vi "Day 4 main.vi"() -> ()   [LabVIEW 2020]
uses:
  bf0b99a3-431b-4a45-be7d-e08dca16cb5f.vi
panel:
  out "Any overlap":i32
  out "Completely overlap":i32
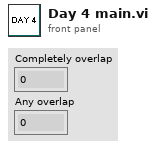
[diagram p1: front panel]
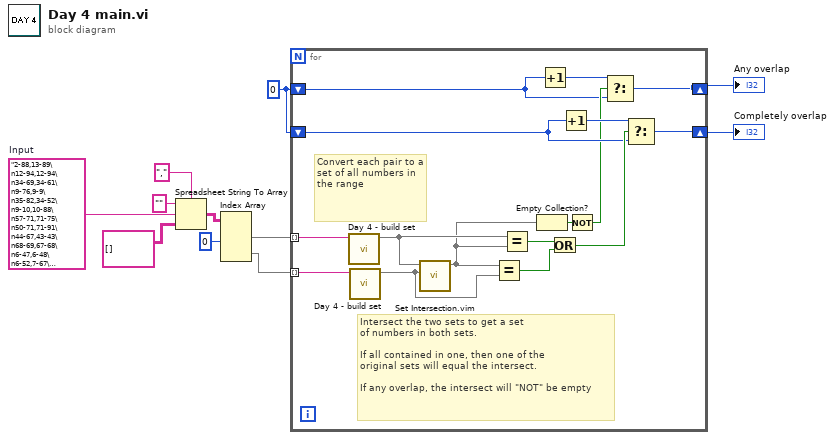
[diagram p0: block diagram]
diagram:
  w2 = 0
  w11 = "2-88,13-89\n12-94,12-94\n34-69,34-61\n9-76,9-9\n35-82,34-52\n9-10,10-88\n57-71,71-75\n50-71,71-91\n44-67,43-43\n68-69,67-68\n6-47,6-48\n6-52,7-67\n43-51,40-44\n56-67,57-69\n94-94,68-94\n10-97,9-9\n40-95,40-98\n22-81,22-22\n7-58,7-59\n8-82,82-82\n22-27,23-44\n5-27,7-28\n11-75,11-75\n7-90,99-99\n65-89,65-66\n24-52,29-53\n41-57,27-58\n14-95,13-26\n27-34,26-75\n18-33,33-56\n21-95,21-95\n20-29,69-71\n81-81,23-90\n47-83,47-82\n28-50,86-98\n50-76,21-50\n3-69,64-79\n17-97,10-16\n54-92,10-93\n7-75,45-77\n72-72,42-73\n13-80,81-87\n25-26,25-64\n38-48,38-38\n2-99,2-99\n48-93,67-92\n12-85,2-94\n14-75,7-82\n29-46,23-29\n50-94,4-51\n3-37,37-91\n24-91,91-91\n25-48,44-47\n2-77,1-26\n1-58,1-21\n16-93,16-93\n3-99,8-98\n23-23,6-23\n17-67,68-68\n4-15,1-4\n35-41,35-40\n6-88,52-89\n11-48,11-61\n4-64,12-65\n7-90,7-8\n1-89,6-73\n64-69,38-70\n26-67,59-66\n41-54,16-42\n2-99,9-96\n2-8,7-88\n12-95,97-97\n17-92,12-93\n27-56,27-28\n19-66,65-77\n1-95,94-94\n24-48,23-95\n40-74,74-74\n20-99,20-97\n60-73,61-74\n23-85,23-86\n37-69,69-69\n37-64,27-37\n7-53,7-27\n84-97,93-94\n26-51,50-52\n12-93,13-93\n28-86,29-29\n11-25,18-46\n97-99,91-98\n27-73,53-58\n25-77,6-26\n26-29,29-68\n11-17,11-28\n99-99,13-99\n70-92,48-92\n50-61,50-62\n2-95,77-94\n17-17,17-90\n95-95,16-95\n12-96,13-97\n28-98,28-28\n18-91,3-80\n1-95,1-19\n86-89,22-89\n37-96,3-96\n2-18,18-56\n8-72,71-73\n46-48,32-47\n57-69,57-78\n10-22,9-9\n6-96,6-6\n44-58,5-59\n6-8,7-93\n76-95,77-99\n97-99,3-98\n69-69,64-69\n38-68,67-96\n68-74,67-95\n20-68,69-69\n6-88,9-85\n47-66,47-55\n9-94,93-95\n19-29,28-89\n4-83,90-90\n2-95,1-95\n36-37,36-36\n12-90,45-68\n1-80,89-94\n95-99,6-96\n1-1,2-95\n47-81,46-80\n1-57,38-47\n5-7,7-98\n18-75,18-94\n39-70,39-70\n62-93,62-62\n30-32,31-54\n22-82,82-84\n83-92,84-98\n54-93,6-94\n74-91,73-90\n11-90,11-90\n92-98,96-97\n13-73,55-69\n47-95,46-95\n11-97,11-99\n53-68,53-53\n45-89,45-46\n99-99,38-89\n14-88,96-96\n6-78,6-7\n31-67,67-67\n96-96,48-96\n40-69,25-39\n10-60,9-61\n38-97,78-93\n52-69,51-60\n21-72,21-33\n24-90,89-90\n36-83,84-84\n44-58,44-68\n95-95,82-94\n13-91,91-95\n27-95,94-96\n60-82,61-83\n11-77,12-12\n7-91,6-90\n15-94,14-48\n5-73,5-74\n10-40,10-40\n59-94,59-93\n84-84,84-84\n8-8,7-75\n20-81,20-81\n5-96,96-99\n5-63,5-6\n2-93,2-93\n72-74,31-73\n6-54,5-47\n8-36,9-86\n1-95,94-94\n11-66,10-73\n45-52,52-99\n1-92,1-95\n76-90,76-77\n6-53,54-55\n44-52,45-95\n5-70,27-70\n3-56,6-55\n28-37,36-37\n54-97,54-98\n4-63,1-4\n5-64,65-65\n19-74,17-18\n12-26,12-12\n34-78,35-99\n42-42,3-42\n69-70,69-77\n49-75,50-95\n30-52,1-28\n25-80,25-25\n97-99,10-98\n36-55,36-54\n6-55,8-55\n60-80,61-81\n76-81,37-77\n19-20,20-20\n11-33,33-85\n31-60,7-32\n3-9,1-2\n40-87,22-40\n9-35,8-35\n9-75,35-75\n19-86,18-85\n33-52,45-53\n15-49,49-66\n40-83,1-41\n10-54,23-88\n83-94,43-83\n7-74,3-75\n18-79,17-18\n6-63,1-6\n19-39,39-77\n69-78,69-79\n14-26,1-23\n3-49,1-58\n39-40,38-39\n16-58,54-57\n34-83,17-34\n79-88,10-80\n73-86,73-86\n4-15,13-14\n6-94,6-6\n84-93,35-84\n56-81,55-81\n3-30,3-4\n5-94,4-96\n5-87,42-87\n98-99,63-79\n20-95,10-21\n40-87,39-41\n39-90,40-97\n20-54,24-88\n1-40,2-65\n57-97,63-96\n1-42,1-1\n5-11,11-66\n39-96,38-95\n5-72,6-73\n7-7,10-96\n97-97,13-97\n71-97,2-4\n79-79,76-79\n20-56,56-74\n57-76,62-68\n20-63,20-57\n19-68,69-69\n41-70,41-70\n37-42,27-44\n77-98,57-99\n18-92,91-96\n10-85,10-96\n43-61,6-44\n25-65,66-95\n12-29,12-80\n22-70,69-71\n77-78,6-77\n20-89,22-88\n79-88,20-88\n98-98,3-99\n58-80,58-66\n27-32,25-47\n80-91,80-95\n24-70,24-86\n52-60,52-62\n80-80,16-80\n3-43,10-88\n2-80,1-99\n34-87,34-88\n28-30,28-32\n13-55,7-55\n16-38,7-16\n25-33,32-77\n58-90,57-57\n7-94,6-7\n5-97,32-96\n71-71,51-71\n10-21,10-11\n3-9,8-98\n26-34,1-81\n35-49,35-50\n11-70,10-71\n25-72,24-99\n27-84,71-72\n50-72,50-71\n11-62,11-34\n93-97,92-96\n71-71,28-71\n72-80,65-81\n27-32,23-28\n31-79,32-79\n12-80,12-81\n38-63,6-39\n27-98,60-97\n45-83,35-45\n52-52,30-52\n11-97,12-14\n3-94,1-99\n4-23,16-22\n1-12,13-91\n14-80,14-78\n3-89,1-3\n28-99,27-87\n14-50,11-66\n40-88,39-39\n38-98,98-99\n5-91,4-91\n4-22,23-23\n20-90,24-91\n2-63,1-62\n14-81,13-80\n52-52,1-51\n8-11,11-93\n9-66,1-9\n44-86,43-68\n13-13,13-94\n40-67,40-68\n70-73,34-68\n5-83,2-11\n37-49,36-49\n11-97,99-99\n44-99,43-98\n50-98,50-97\n38-39,38-80\n83-83,2-84\n14-40,3-23\n41-94,41-96\n61-83,59-62\n22-95,22-96\n32-77,32-77\n22-97,23-96\n39-85,70-84\n4-95,3-95\n14-39,14-38\n9-68,68-96\n62-63,3-48\n21-25,22-90\n4-4,3-98\n85-89,85-99\n7-42,7-43\n31-82,82-84\n45-53,41-54\n38-66,37-66\n5-80,4-72\n1-1,2-97\n3-3,2-3\n47-61,42-61\n70-94,94-98\n1-51,1-51\n53-70,93-99\n43-72,72-82\n3-7,6-77\n71-95,82-92\n82-89,6-82\n3-43,4-76\n45-91,46-91\n12-87,13-87\n11-92,11-46\n3-73,3-72\n91-91,47-92\n12-93,14-94\n43-45,9-44\n10-87,11-87\n20-34,33-88\n48-71,15-97\n20-64,19-64\n3-57,57-57\n6-7,7-99\n4-19,19-96\n68-72,69-72\n14-45,14-14\n22-93,22-23\n8-34,8-15\n83-93,92-96\n11-94,12-94\n54-84,38-85\n93-98,3-55\n32-77,39-40\n3-15,15-93\n16-28,11-29\n1-95,94-96\n6-25,25-26\n32-96,99-99\n1-35,2-5\n73-91,65-74\n62-77,41-63\n72-72,72-93\n5-81,5-81\n81-83,32-81\n68-89,68-89\n30-35,30-61\n48-97,8-49\n85-94,12-94\n15-95,15-96\n4-98,3-4\n33-84,33-92\n28-58,29-59\n44-80,44-80\n11-84,83-83\n95-98,1-96\n3-44,21-43\n91-91,46-69\n91-98,1-90\n3-20,19-72\n3-92,4-55\n23-68,98-98\n26-97,80-83\n98-98,2-97\n30-92,74-92\n6-44,7-60\n18-23,36-47\n9-94,98-99\n11-20,11-75\n50-95,5-51\n13-83,20-84\n27-27,27-47\n95-96,56-95\n27-28,27-29\n31-95,31-31\n19-50,21-23\n19-48,30-55\n7-36,22-80\n3-5,6-99\n21-22,23-52\n3-70,3-70\n4-8,7-90\n28-60,60-98\n81-93,58-82\n2-6,3-16\n15-75,16-76\n8-86,6-6\n1-78,78-95\n37-91,37-99\n94-94,17-94\n53-80,80-81\n1-90,89-89\n21-32,21-73\n65-74,65-74\n24-54,89-92\n8-47,9-47\n8-36,12-41\n6-79,1-23\n79-83,24-84\n91-91,16-92\n14-84,14-15\n51-67,50-50\n6-93,96-96\n29-55,29-43\n36-37,36-77\n36-36,19-35\n84-84,60-89\n66-88,14-89\n14-69,28-93\n79-94,39-62\n85-89,89-89\n1-78,2-78\n44-52,42-53\n55-97,55-97\n32-81,74-80\n90-90,16-89\n3-96,2-37\n15-58,16-71\n5-93,6-93\n1-4,4-13\n61-96,61-99\n17-87,17-86\n34-48,35-49\n17-58,10-17\n1-11,12-68\n56-86,27-64\n73-80,73-77\n96-96,76-97\n23-32,23-31\n3-94,5-95\n67-98,66-72\n87-93,56-92\n4-15,5-15\n24-76,25-75\n43-59,33-60\n66-74,66-68\n18-90,17-57\n68-72,72-93\n6-19,19-29\n94-99,6-95\n20-85,10-21\n45-66,45-67\n73-74,12-73\n35-75,34-59\n67-88,80-88\n99-99,2-97\n15-90,14-14\n9-59,9-86\n18-52,52-79\n65-73,27-74\n89-96,88-96\n97-97,5-78\n92-94,48-93\n27-40,27-57\n7-95,1-8\n7-17,7-49\n66-66,65-89\n7-46,12-78\n15-29,15-38\n7-7,8-64\n13-22,13-21\n11-11,10-45\n84-84,30-84\n42-91,91-91\n65-87,29-87\n87-87,18-86\n17-66,17-65\n87-88,78-86\n57-57,58-87\n22-53,22-54\n8-62,7-62\n37-90,37-91\n50-86,49-86\n6-58,6-67\n32-60,32-63\n91-96,91-91\n13-94,13-14\n4-95,4-95\n1-86,4-87\n30-96,59-95\n10-28,8-59\n2-49,66-71\n96-99,4-97\n3-74,2-2\n29-76,75-75\n4-92,4-91\n16-94,14-16\n35-35,36-96\n39-67,66-66\n17-97,16-67\n1-99,46-98\n41-74,40-74\n45-68,45-69\n68-95,94-99\n14-51,13-31\n91-91,4-91\n46-66,2-67\n61-66,6-71\n66-69,55-89\n11-11,6-10\n72-91,73-94\n1-92,1-16\n25-98,35-74\n56-87,73-87\n57-59,1-58\n4-5,4-91\n27-31,30-68\n98-98,22-98\n28-95,84-94\n9-24,8-24\n21-30,22-38\n79-81,6-83\n34-96,34-83\n31-33,26-32\n36-59,50-52\n25-95,19-25\n97-97,75-90\n97-99,27-98\n7-48,32-52\n12-72,11-33\n3-41,3-41\n2-95,3-95\n71-71,52-72\n92-98,20-92\n14-90,15-99\n86-97,85-87\n44-71,44-71\n10-68,1-10\n47-77,11-46\n8-25,25-47\n22-34,25-34\n17-90,18-48\n31-94,30-94\n10-97,10-96\n21-44,22-97\n42-97,2-98\n84-91,50-85\n60-96,78-82\n81-85,73-80\n41-73,40-73\n48-65,47-56\n5-42,6-79\n33-33,33-83\n46-79,47-79\n61-91,23-92\n93-95,3-94\n32-43,31-51\n83-97,70-83\n24-93,94-94\n2-94,8-91\n45-61,46-65\n46-50,48-75\n23-95,57-84\n3-99,92-95\n85-85,2-61\n42-87,87-93\n95-99,2-96\n3-4,3-98\n1-87,7-87\n34-72,72-73\n11-84,8-12\n80-99,63-98\n96-99,7-97\n73-75,30-73\n60-87,7-61\n21-41,19-40\n14-77,76-86\n53-97,36-98\n34-54,33-54\n4-36,11-66\n6-10,10-94\n1-57,3-87\n15-39,16-39\n34-72,14-33\n1-3,3-93\n23-53,22-53\n24-44,23-34\n9-28,3-9\n12-99,99-99\n87-98,87-98\n11-11,11-73\n96-96,4-91\n91-91,8-92\n18-47,18-94\n57-59,27-59\n12-96,13-75\n1-27,26-61\n21-60,60-61\n30-67,31-67\n22-78,22-78\n6-77,7-52\n28-45,44-78\n34-87,90-94\n65-76,77-77\n11-76,57-58\n83-84,14-83\n70-97,11-70\n97-98,11-97\n29-29,16-29\n87-94,18-87\n53-71,70-70\n3-96,2-90\n11-80,13-99\n68-68,69-83\n64-97,1-98\n39-42,40-58\n35-49,35-49\n58-88,58-87\n67-67,13-66\n20-20,6-19\n16-67,16-17\n3-46,2-4\n41-96,41-88\n20-89,18-21\n4-84,4-84\n81-82,20-81\n94-94,28-93\n64-74,8-65\n3-73,5-36\n15-67,6-86\n33-33,32-91\n23-97,57-97\n8-58,8-46\n9-10,9-99\n67-93,69-92\n93-99,5-93\n95-96,95-98\n15-22,35-53\n55-97,38-98\n95-99,3-96\n12-12,12-62\n89-89,41-88\n9-10,9-92\n41-85,67-84\n10-97,2-11\n19-73,61-72\n38-79,78-80\n49-61,50-72\n70-71,71-72\n25-32,26-31\n2-5,3-62\n12-94,11-93\n26-95,27-98\n40-81,40-80\n34-71,34-95\n99-99,16-89\n14-93,93-96\n19-70,4-20\n7-28,1-29\n13-59,12-59\n44-97,11-45\n8-36,36-37\n94-95,7-94\n43-43,9-42\n16-98,3-13\n89-96,59-82\n9-50,9-51\n70-98,69-97\n84-87,84-87\n25-83,13-70\n63-71,62-71\n3-31,3-96\n53-67,13-76\n98-98,59-99\n4-39,5-40\n19-91,17-90\n28-50,36-45\n34-86,33-38\n58-80,57-80\n90-90,9-90\n98-98,37-72\n2-39,3-53\n85-97,28-84\n96-97,86-98\n38-78,30-39\n1-42,2-41\n7-28,8-27\n6-74,7-75\n85-87,49-86\n98-98,16-46\n42-90,41-70\n5-70,6-70\n13-75,75-75\n25-69,5-51\n13-43,2-14\n77-91,78-78\n17-97,16-18\n3-94,1-3\n33-86,32-92\n13-57,57-68\n18-88,19-95\n11-97,11-96\n17-67,17-67\n44-95,44-94\n21-85,20-85\n30-64,41-64\n34-68,35-68\n37-77,77-79\n96-97,9-96\n78-85,9-79\n80-80,35-79\n16-50,16-36\n65-85,7-85\n52-92,2-52\n77-77,30-78\n4-61,2-5\n41-91,30-90\n93-96,20-90\n9-11,10-73\n39-42,38-42\n46-72,45-76\n57-63,56-66\n9-68,5-46\n5-92,98-98\n39-46,39-46\n10-48,10-65\n3-22,7-91\n43-82,2-94\n21-69,20-69\n70-70,2-71\n9-94,8-91\n23-99,23-80\n6-98,6-97\n45-45,22-44\n31-79,32-32\n47-67,47-48\n5-80,80-81\n34-54,29-55\n16-97,16-96\n6-71,71-74\n17-47,17-46\n74-85,85-86\n7-10,9-82\n30-30,30-90\n51-54,55-55\n20-28,21-98\n67-67,64-66\n50-51,35-50\n4-68,5-5\n1-4,4-40\n20-20,20-84\n29-31,26-73\n12-12,11-12\n45-94,44-93\n36-45,18-37\n14-41,13-98\n38-42,42-84\n32-63,31-62\n32-79,1-79\n32-32,32-88\n83-95,83-96\n50-84,49-83\n30-56,30-74\n7-67,67-82\n5-39,40-94\n3-7,7-82\n42-45,42-67\n1-97,96-99\n30-87,30-64\n3-97,3-98\n52-81,52-81\n65-80,65-80\n46-55,54-91\n17-88,87-92\n7-97,97-97\n57-81,57-81\n54-97,54-54\n13-13,13-86\n30-35,36-36\n77-77,68-76\n11-82,12-91\n7-72,2-48\n85-94,28-86\n17-88,88-99\n9-56,7-9\n56-96,33-96\n85-89,85-89\n13-13,13-99\n76-93,62-76\n86-86,31-86\n31-95,31-96\n68-70,44-69\n9-54,9-10\n66-97,25-98\n44-93,93-93\n63-63,17-62\n3-98,2-10\n18-96,19-97\n19-80,2-81\n44-45,4-44\n1-37,7-36\n59-61,39-62\n33-98,33-57\n38-77,37-76\n13-96,11-14\n28-98,29-99\n4-44,2-45\n37-95,37-95\n53-68,54-68\n3-72,4-88\n14-21,21-82\n43-65,42-47\n21-52,51-93\n65-79,56-65\n22-65,36-77\n42-54,53-99\n10-95,9-95\n1-78,2-76\n81-81,16-81\n26-49,29-70\n45-87,44-87\n14-15,14-67\n14-15,14-84\n2-42,41-79\n1-93,93-94\n61-98,60-97\n3-9,12-99\n48-62,49-56\n64-65,41-64\n27-52,27-51\n88-91,30-89\n17-46,46-46\n10-80,11-81\n3-7,1-6\n80-81,80-96\n67-96,67-96\n96-98,2-96\n89-90,60-89\n16-83,16-82\n67-77,68-70\n33-68,33-37\n8-29,1-7\n28-71,28-70\n64-89,79-89\n18-35,18-36\n20-86,20-88\n68-69,40-68\n24-74,23-82\n79-88,79-88\n5-56,4-55\n1-98,2-2\n10-99,4-24\n12-15,13-15\n30-93,99-99\n6-14,6-97\n3-86,4-52\n15-52,13-52\n28-78,78-79\n27-28,27-95\n40-88,29-96\n1-3,2-52\n27-43,27-33\n23-65,54-99\n4-49,48-50\n46-67,47-68\n94-94,2-94\n24-31,30-66\n14-87,6-58\n2-5,4-98\n40-92,39-91\n2-87,87-88\n7-74,19-73\n58-91,58-92\n11-82,5-97\n62-65,4-62\n95-96,8-95\n6-68,6-68\n5-98,4-10\n46-72,89-96\n24-58,58-92\n33-36,37-94\n47-48,48-76\n18-20,3-32\n11-65,10-58\n32-97,32-95\n27-53,19-75\n10-60,45-59\n32-62,63-65\n1-88,2-88\n48-93,63-92\n46-79,78-96\n18-47,4-17\n6-63,6-7\n39-80,36-69\n20-78,20-78\n26-81,26-27\n23-96,20-79\n45-59,45-60\n37-47,36-64\n33-45,5-42\n3-98,4-98\n18-75,4-19\n10-93,10-10\n24-70,7-24\n20-53,40-49\n56-81,72-80\n1-70,4-71\n15-18,19-92\n84-98,83-95\n35-48,47-49\n27-63,62-78\n9-79,14-95\n5-77,4-77\n20-39,20-40\n26-67,72-92\n69-80,55-80\n68-83,68-92\n87-87,6-86\n1-92,1-94\n14-81,14-99\n49-51,49-52\n71-71,49-70\n69-70,69-72\n18-54,3-50\n97-99,1-97\n4-34,33-33\n67-84,11-84\n31-52,47-51\n81-97,97-98\n27-62,54-61\n1-83,1-99\n30-78,30-78\n12-38,12-37\n37-76,24-74\n1-96,1-95\n96-96,12-96\n41-61,40-60\n81-87,81-99\n1-19,9-19\n2-8,7-42\n35-36,36-71\n67-79,67-78\n69-69,65-68\n8-8,9-64\n4-12,6-78\n14-47,47-64\n9-93,9-93\n95-98,15-29\n30-87,88-88\n12-77,78-78\n8-15,18-50\n10-98,11-97\n1-2,1-97\n2-92,2-86\n50-50,50-87"  # Input
  n1 = Spreadsheet String To Array(delimiter (Tab)=",", format string="", spreadsheet string=w11, array type (2D Dbl)=string[][] []) -> (array=w7:string[][])
  n2 = Index Array(array=w7, index (col) #1=0 ("disabled index (col)")) -> (element #1=w5:string[], element #2=w4:string[])  [unwired: 3 in]
  n3 = for {
    tunnel: w5 -> [w13] mode=indexing
    tunnel: w4 -> [w12] mode=indexing
    shift-right: [w23] -> w3
    shift-left: w2 -> [w20]
    shift-right: [w15] -> w1
    shift-left: w2 -> [w14]
    # "Intersect the two sets to get a set\nof numbers in both sets.\n\nIf all contained in one, then one of the \noriginal sets will equal the intersect.\n\nIf any overlap, the intersect will \"NOT\" be empty"
    # "Convert each pair to a set of all numbers in the range"
    n4 = call "Day 4 - build set.vi"("String (a-b)"=w13) -> ("Set (a..b inclusive)"=w27:set{i32})  [unwired: 10 in]
    n5 = call "Day 4 - build set.vi"("String (a-b)"=w12) -> ("Set (a..b inclusive)"=w26:set{i32})  [unwired: 10 in]
    n6 = call "Set Intersection.vim"("set 2"=w26, "set 1"=w27) -> ("intersection"=w19:set{i32})  [unwired: 9 in]
    n7 = Equal?(x=w19, y=w26) -> (x = y?=w24:bool)
    n8 = Equal?(x=w27, y=w19) -> (x = y?=w25:bool)
    n9 = Empty Collection?(1:w19) -> (0:w18:bool)
    n10 = Increment(x=w14) -> (x+1=w17:i32)
    n11 = Or(x=w25, y=w24) -> (x .or. y?=w22:bool)
    n12 = Increment(x=w20) -> (x+1=w21:i32)
    n13 = Not(x=w18) -> (.not. x?=w16:bool)
    n14 = Select(t=w17, s=w16, f=w14) -> (s? t:f=w15:i32)
    n15 = Select(t=w21, s=w22, f=w20) -> (s? t:f=w23:i32)
  }
  "Completely overlap" <- w3
  "Any overlap" <- w1
